vi "Get alpha n.vi"(10 "n":i32, 11 "Analytical Serial Arm Class in":refnum<class "NI_Robotics_Analytical Serial Arm Class.lvclass">) -> (2 "alpha n":dbl, 3 "Analytical Serial Arm Class out":refnum<class "NI_Robotics_Analytical Serial Arm Class.lvclass">)   [LabVIEW 2017, in "NI_Robotics_Analytical Serial Arm Class.lvclass"]
uses:
  <vilib>/robotics/Kinematics/Analytical/Generic/NI_Robotics_Analytical Serial Arm Class.lvclass
  c:/Program Files (x86)/National Instruments/LabVIEW 2017/vi.lib/robotics/Kinematics/Robot/NI_Robotics_Serial Robot Arm.lvclass
  <vilib>/robotics/Kinematics/Link/NI_Robotics_Link.lvclass/NI_Robotics_Link.ctl
  <vilib>/robotics/Kinematics/Robot/NI_Robotics_Serial Robot Arm.lvclass
  <vilib>/robotics/Kinematics/Link/NI_Robotics_Link.lvclass
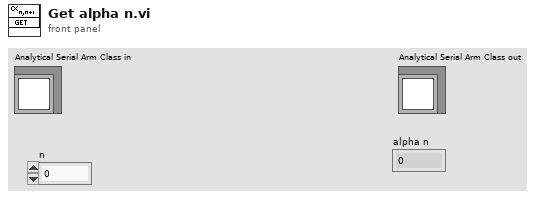
[diagram p1: front panel]
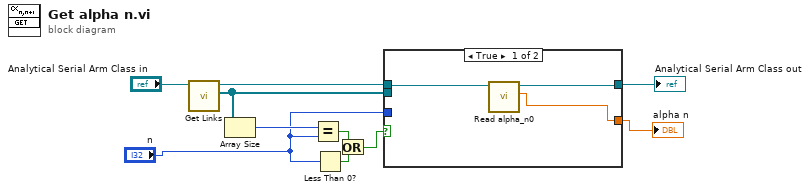
[diagram p0: block diagram]
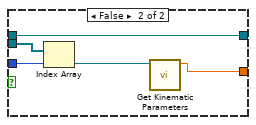
[diagram p2: hidden frame]
diagram:
  n1 = call <vilib>:"Get Links.vi"("serial arm in"="Analytical Serial Arm Class in") -> ("links"=w9:refnum<class "NI_Robotics_Link.lvclass">[], "serial arm out"=w8:refnum<class "NI_Robotics_Analytical Serial Arm Class.lvclass">)  [unwired: 8 in, 1 out]
  n2 = Array Size(array=w9) -> (size(s)=w5:i32)
  n3 = Equal?(x=w5, y="n") -> (x = y?=w3:bool)
  n4 = Less Than 0?(x="n") -> (x < 0?=w2:bool)
  n5 = Or(x=w3, y=w2) -> (x .or. y?=w4:bool)
  n6 = case shown="True" w4 {
    tunnel: w9 -> [_ w17]
    tunnel: [w13 w15] -> w6
    tunnel: w8 -> [w11 w16]
    tunnel: [w12 w16] -> w7
    tunnel: "n" -> [_ w14]
    frame True {
      n7 = call <vilib>:"Read alpha_n0.vi"("Analytical Serial Arm Class in"=w11) -> ("alpha_n0"=w13:dbl, "Analytical Serial Arm Class out"=w12:refnum<class "NI_Robotics_Analytical Serial Arm Class.lvclass">)  [unwired: 8 in, 1 out]
    }
    frame False {
      n8 = Index Array(array=w17, index=w14) -> (element=w18:refnum<class "NI_Robotics_Link.lvclass">)
      n9 = call <vilib>:"Get Kinematic Parameters.vi"("NI_Robotics_Link in"=w18) -> ("Twist Angle"=w15:dbl)  [unwired: 6 in, 4 out]
    }
  }
  "alpha n" <- w6
  "Analytical Serial Arm Class out" <- w7
